vi "Build.vi"() -> ()   [LabVIEW 2015]
uses:
  <vilib>/Utility/sysdir.llb/System Directory Type.ctl
  <vilib>/AppBuilder/AB_API_Simple/Build (path).vi
  <vilib>/AppBuilder/AB_API_Simple/NI_App_Builder_API.lvlib
panel:
  out "errors":errorcluster[](array[cluster])
  out "return code":i32
  out "args":string[][](array[string])
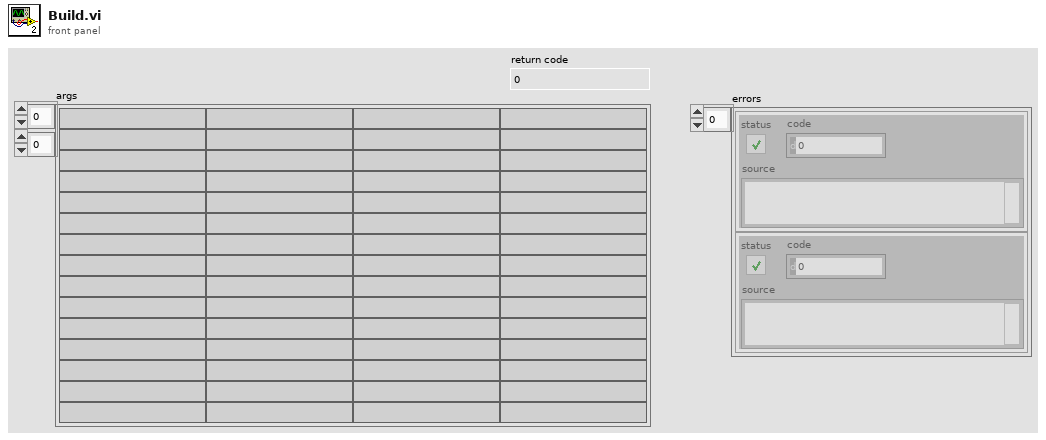
[diagram p1: front panel]
types:
  T1 = enum32{"Invalid", "Standard", "Closed", "Hidden", "Minimized", "Maximized"}
  T2 = enum16{"open", "replace", "create", "open or create", "replace or create", "replace or create with confirmation"}
  T3 = typedef "System Directory Type.ctl" = i32
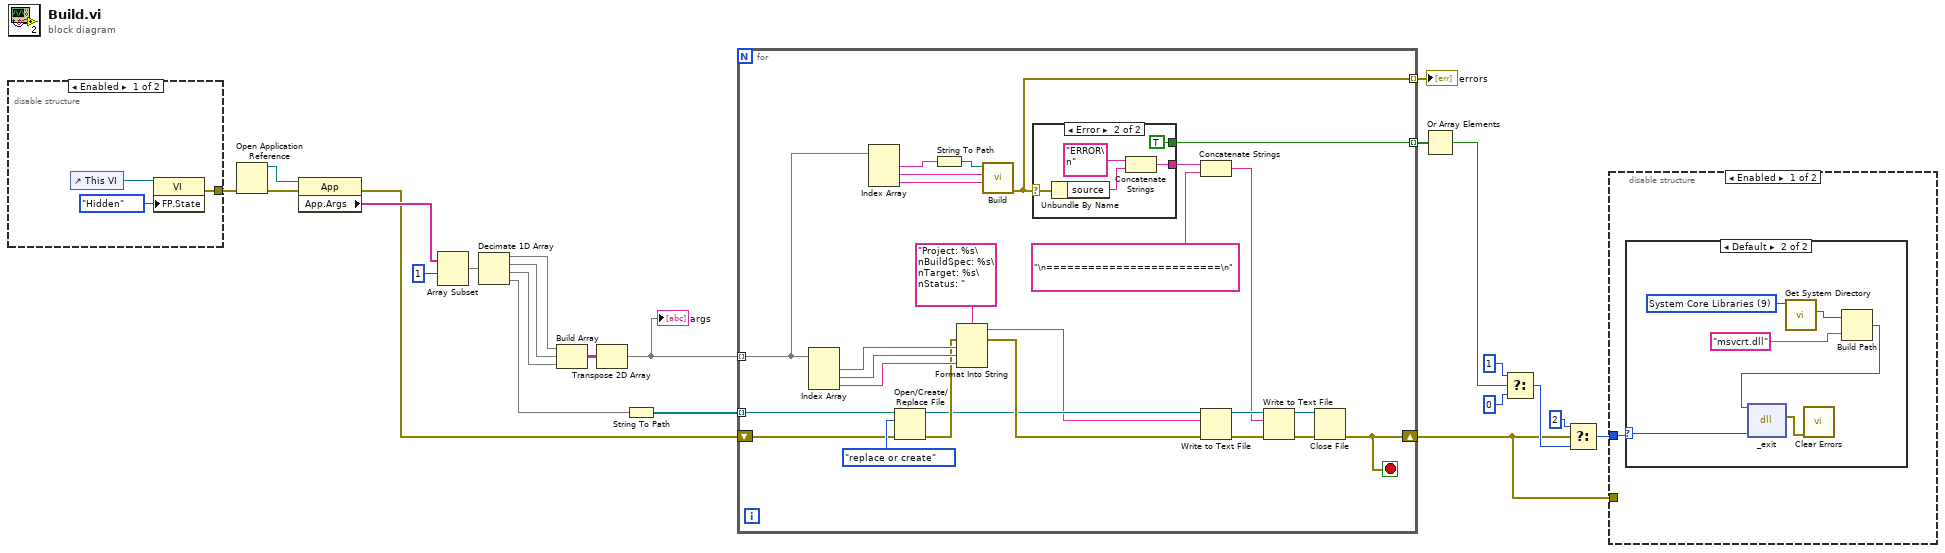
[diagram p0: block diagram]
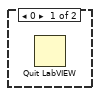
[diagram p3: hidden frame]
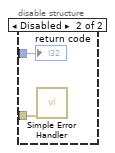
[diagram p4: hidden frame]
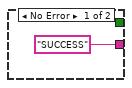
[diagram p5: hidden frame]
diagram:
  n1 = disable-structure shown="Enabled" {
    disable-tunnel: [w24 _] -> w21
    frame Enabled {
      n2 = control-ref of="This VI"() -> (w26:refnum<vi>)
      n3 = property class="VI"(reference=w26, "FP.State"=T1."Hidden" ("Front Panel Window:State")) -> (error out=w24:errorcluster)  [unwired: 1 in, 1 out]
    }
    frame Disabled {
    }
  }
  n4 = Open Application Reference(8:w21) -> (0:w22:errorcluster, 3:w23:refnum<vi>)  [unwired: 3 in]
  n5 = property class="App"(reference=w23, error in=w22) -> (error out=w5:errorcluster, "App.Args"=w6:string[])  [unwired: 1 out]
  n6 = Array Subset(array=w6, index=1) -> (w19:string[])  [unwired: 1 in]
  n7 = Decimate 1D Array(w19) -> (w4:string[], w11:string[], w10:string[], w1:string[])
  n8 = Build Array(w4, w11, w10) -> (w8:string[][])
  n9 = Transpose 2D Array(2D array=w8) -> (transposed array=w7:string[][])
  "args" <- w7
  n10 = String To Path(string=w1) -> (path=w3:path[])
  n11 = for {
    shift-right: [w37] -> w2
    shift-left: w5 -> [w28]
    tunnel: [w46] -> w18 mode=indexing
    tunnel: w7 -> [w40] mode=indexing
    tunnel: [w42] -> w9 mode=indexing
    tunnel: w3 -> [w27] mode=indexing
    stop <- w37 stop-if-true
    n12 = Index Array(array=w40) -> (element #1=w36:string, element #2=w35:string, element #3=w34:string)  [unwired: 3 in]
    n13 = Index Array(array=w40) -> (element #1=w45:string, element #2=w44:string, element #3=w43:string)  [unwired: 3 in]
    n14 = Open/Create/Replace File(file path (use dialog)=w27, error in=w28, operation (0:open)=T2."replace or create") -> (refnum out=w30:refnum<file>, error out=w32:errorcluster)  [unwired: 3 in, 1 out]
    n15 = String To Path(string=w45) -> (path=w52:path)
    n16 = Format Into String(format string="Project: %s\nBuildSpec: %s\nTarget: %s\nStatus: ", error in=w32, w36, w35, w34) -> (resulting string=w29:string, error out=w31:errorcluster)  [unwired: 1 in]
    n17 = call-poly <vilib>:"Build.vi"("Name of target (My Computer)"=w43, "Name of build specification (if empty: build all)"=w44, "Path to project"=w52) -> ("error out"=w42:errorcluster)  [unwired: 7 in, 1 out]
    n18 = case shown="Error" w42 {
      selector: w42 -> [_ w56]
      tunnel: ["SUCCESS" ("format string") w55] -> w51
      tunnel: [_ TRUE] -> w46
      frame No Error {
      }
      frame Error {
        n19 = Unbundle By Name(w56) -> ("source"=w57:string)
        n20 = Concatenate Strings("ERROR\n" ("format string"), w57) -> (w55:string)
      }
    }
    n21 = Concatenate Strings(w51, "\n=========================\n" ("format string")) -> (w47:string)
    n22 = Write to Text File(file (use dialog)=w30, text=w29, error in=w31) -> (refnum out=w48:refnum<file>, error out=w49:errorcluster)  [unwired: 1 in, 1 out]
    n23 = Write to Text File(file (use dialog)=w48, text=w47, error in=w49) -> (refnum out=w38:refnum<file>, error out=w39:errorcluster)  [unwired: 1 in, 1 out]
    n24 = Close File(refnum=w38, error in=w39) -> (error out=w37:errorcluster)  [unwired: 1 out]
  }
  "errors" <- w9
  n25 = Or Array Elements(Boolean array=w18) -> (logical OR=w17:bool)
  n26 = Select(t=1 ("code"), s=w17, f=0 ("code")) -> (s? t:f=w15:i32)
  n27 = Select(t=2 ("code"), s=w2, f=w15) -> (s? t:f=w12:i32)
  n28 = disable-structure shown="Enabled" {
    disable-tunnel: w12 -> [w59 w67]
    disable-tunnel: w2 -> [_ w66]
    frame Enabled {
      n29 = case shown="Default" w59 {
        selector: w59 -> [_ w65]
        frame 0 {
          n30 = Quit LabVIEW() -> ()  [unwired: 1 in]
        }
        frame Default {
          w61 = T3 9 items=["User Home"=0, "User Desktop"=1, "User Documents"=2, "User Application Data"=3, "User Preferences"=4, "User Temporary"=5, "Public Documents"=6, "Public Application Data"=7, "Public Preferences"=8, "Public Cache"=13, "System Core Libraries"=9, "System Installed Libraries"=10, "Application Files"=11, "Boot Volume Root"=12] ("system directory type")
          n31 = call <vilib>:"Get System Directory.vi"("system directory type"=w61) -> ("system directory"=w62:path)  [unwired: 10 in]
          n32 = Build Path(base path=w62, name or relative path="msvcrt.dll") -> (appended path=w60:path)
          n33 = dll-call lib="C:/Windows/System32/msvcrt.dll" fn="_exit"(path in=w60, "code"=w65) -> (error out=w64:errorcluster)  [unwired: 4 in, 1 out]
          n34 = call <vilib>:"Clear Errors.vi"("error in (no error)"=w64) -> ()  [unwired: 5 in, 2 out]
        }
      }
    }
    frame Disabled {
      n35 = call <vilib>:"Simple Error Handler.vi"("error in (no error)"=w66) -> ()  [unwired: 4 in, 5 out]
      "return code" <- w67
    }
  }
